vi "remining pieces types.vi"(10 "cnt":i32, 11 "Type":enum16{"Z", "I", "O", "S", "L", "J", "T", "N"}(ring)) -> (3 "Type required":enum16{"Z", "I", "O", "S", "L", "J", "T", "N"}(ring))   [LabVIEW 2018]
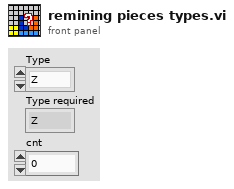
[diagram p1: front panel]
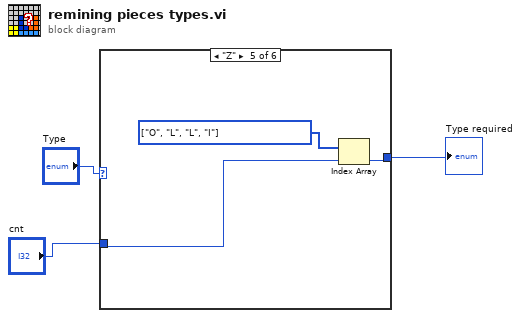
[diagram p0: block diagram]
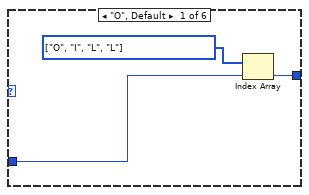
[diagram p2: hidden frame]
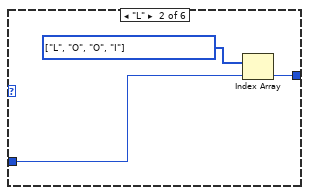
[diagram p3: hidden frame]
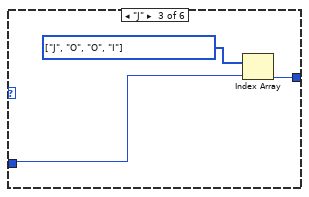
[diagram p4: hidden frame]
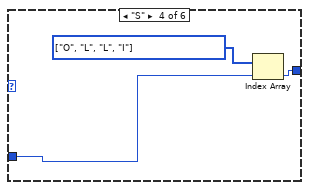
[diagram p5: hidden frame]
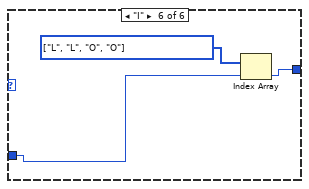
[diagram p6: hidden frame]
diagram:
  n1 = case shown="\"Z\"" "Type" {
    tunnel: "cnt" -> [w5 w8 w10 w13 w17 w20]
    tunnel: [w4 w7 w11 w14 w16 w19] -> w1
    frame "O", Default {
      w6 = enum16{"Z", "I", "O", "S", "L", "J", "T", "N"}[] [enum."O", enum."I", enum."L", enum."L"] items=["Z", "I", "O", "S", "L", "J", "T", "N"] ("Type 2")
      n2 = Index Array(array=w6, index=w5) -> (element=w4:enum16{"Z", "I", "O", "S", "L", "J", "T", "N"})
    }
    frame "L" {
      w9 = enum16{"Z", "I", "O", "S", "L", "J", "T", "N"}[] [enum."L", enum."O", enum."O", enum."I"] items=["Z", "I", "O", "S", "L", "J", "T", "N"] ("Type 2")
      n3 = Index Array(array=w9, index=w8) -> (element=w7:enum16{"Z", "I", "O", "S", "L", "J", "T", "N"})
    }
    frame "J" {
      w12 = enum16{"Z", "I", "O", "S", "L", "J", "T", "N"}[] [enum."J", enum."O", enum."O", enum."I"] items=["Z", "I", "O", "S", "L", "J", "T", "N"] ("Type 2")
      n4 = Index Array(array=w12, index=w10) -> (element=w11:enum16{"Z", "I", "O", "S", "L", "J", "T", "N"})
    }
    frame "S" {
      w15 = enum16{"Z", "I", "O", "S", "L", "J", "T", "N"}[] [enum."O", enum."L", enum."L", enum."I"] items=["Z", "I", "O", "S", "L", "J", "T", "N"] ("Type 2")
      n5 = Index Array(array=w15, index=w13) -> (element=w14:enum16{"Z", "I", "O", "S", "L", "J", "T", "N"})
    }
    frame "Z" {
      w18 = enum16{"Z", "I", "O", "S", "L", "J", "T", "N"}[] [enum."O", enum."L", enum."L", enum."I"] items=["Z", "I", "O", "S", "L", "J", "T", "N"] ("Type 2")
      n6 = Index Array(array=w18, index=w17) -> (element=w16:enum16{"Z", "I", "O", "S", "L", "J", "T", "N"})
    }
    frame "I" {
      w21 = enum16{"Z", "I", "O", "S", "L", "J", "T", "N"}[] [enum."L", enum."L", enum."O", enum."O"] items=["Z", "I", "O", "S", "L", "J", "T", "N"] ("Type 2")
      n7 = Index Array(array=w21, index=w20) -> (element=w19:enum16{"Z", "I", "O", "S", "L", "J", "T", "N"})
    }
  }
  "Type required" <- w1
